vi "main.vi"() -> ()   [LabVIEW 2020]
uses:
  Newport.XPS.CommandInterface
panel:
  out "GatheringStopAndSave":i32
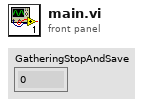
[diagram p1: front panel]
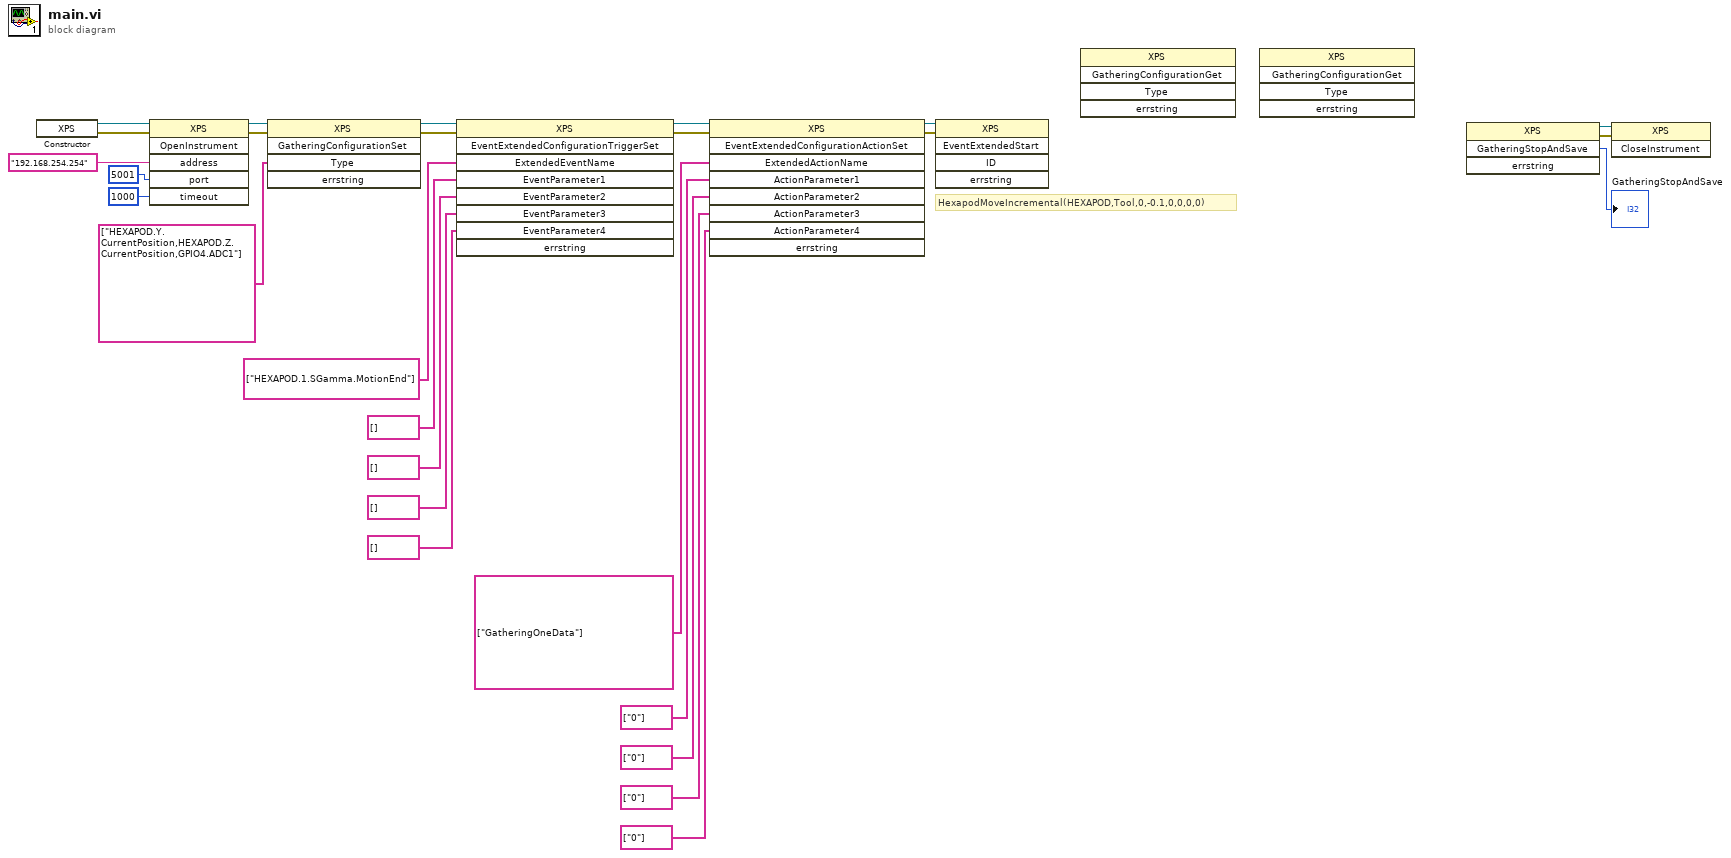
[diagram p0: block diagram]
diagram:
  # "HexapodMoveIncremental(HEXAPOD,Tool,0,-0.1,0,0,0,0)"
  n1 = constructor class="XPS"() -> (reference out=w2:refnum<k24>, error out=w1:errorcluster)  [unwired: 3 in, 1 out]
  n2 = invoke on="Nœud de méthode" class="XPS" method="OpenInstrument"(reference=w2, error in=w1, "address"="192.168.254.254", "port"=5001, "timeout"=1000) -> (reference out=w12:refnum<k24>, error out=w11:errorcluster)  [unwired: 1 in, 4 out]
  n3 = invoke on="Nœud de méthode" class="XPS" method="GatheringConfigurationSet"(reference=w12, error in=w11, "Type"=string[] ["HEXAPOD.Y.CurrentPosition,HEXAPOD.Z.CurrentPosition,GPIO4.ADC1"]) -> (reference out=w10:refnum<k24>, error out=w9:errorcluster)  [unwired: 2 in, 3 out]
  n4 = invoke on="Nœud de méthode" class="XPS" method="EventExtendedConfigurationTriggerSet"(reference=w10, error in=w9, "ExtendedEventName"=string[] ["HEXAPOD.1.SGamma.MotionEnd"], "EventParameter1"=string[] [], "EventParameter2"=string[] [], "EventParameter3"=string[] [], "EventParameter4"=string[] []) -> (reference out=w8:refnum<k24>, error out=w7:errorcluster)  [unwired: 2 in, 7 out]
  n5 = invoke on="Nœud de méthode" class="XPS" method="EventExtendedConfigurationActionSet"(reference=w8, error in=w7, "ExtendedActionName"=string[] ["GatheringOneData"], "ActionParameter1"=string[] ["0"], "ActionParameter2"=string[] ["0"], "ActionParameter3"=string[] ["0"], "ActionParameter4"=string[] ["0"]) -> (reference out=w6:refnum<k24>, error out=w5:errorcluster)  [unwired: 2 in, 7 out]
  n6 = invoke on="Nœud de méthode" class="XPS" method="EventExtendedStart"(reference=w6, error in=w5) -> ()  [unwired: 3 in, 5 out]
  n7 = invoke on="Nœud de méthode" class="XPS" method="GatheringConfigurationGet"() -> ()  [unwired: 5 in, 5 out]
  n8 = invoke on="Nœud de méthode" class="XPS" method="GatheringConfigurationGet"() -> ()  [unwired: 5 in, 5 out]
  n9 = invoke on="Nœud de méthode" class="XPS" method="GatheringStopAndSave"() -> (reference out=w3:refnum<k24>, error out=w4:errorcluster, "GatheringStopAndSave"=→"GatheringStopAndSave":i32)  [unwired: 4 in, 1 out]
  n10 = invoke on="Nœud de méthode" class="XPS" method="CloseInstrument"(reference=w3, error in=w4) -> ()  [unwired: 1 in, 3 out]
